vi "SetGantrySetpoint.vi"(11 "Buttons":bool[](array[boolean])) -> ()   [LabVIEW 2014]
uses:
  Gantry/GantryGlobals.vi
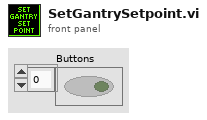
[diagram p1: front panel]
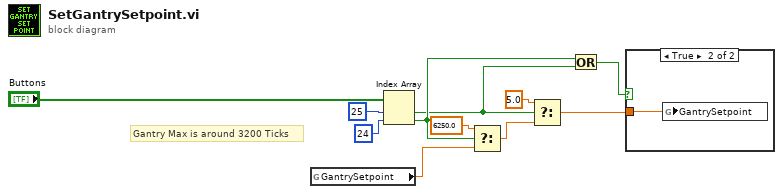
[diagram p0: block diagram]
diagram:
  # "Gantry Max is around 3200 Ticks"
  n1 = global read "GantryGlobals.vi" "GantrySetpoint"() -> (w8:dbl)
  n2 = Index Array(array="Buttons", index #1=25 ("index"), index #2=24 ("index")) -> (element #1=w9:bool, element #2=w10:bool)
  n3 = Select(t=6250.0, s=w10, f=w8) -> (s? t:f=w1:dbl)
  n4 = Select(t=5.0, s=w9, f=w1) -> (s? t:f=w7:dbl)
  n5 = Or(x=w10, y=w9) -> (x .or. y?=w11:bool)
  n6 = case shown="True" w11 {
    tunnel: w7 -> [_ w12]
    frame False {
    }
    frame True {
      n7 = global write "GantryGlobals.vi" "GantrySetpoint"(w12) -> ()
    }
  }
